vi "Handle WELCOME.vi"(8 "error in (no error)":errorcluster, 9 "WAMP Message":T1 {"Message Codes" items=["HELLO"=1, "WELCOME"=2, "ABORT"=3, "GOODBYE"=6, "ERROR"=8, "PUBLISH"=16, "PUBLISHED"=17, "SUBSCRIBE"=32, "SUBSCRIBED"=33, "UNSUBSCRIBE"=34, "UNSUBSCRIBED"=35, "EVENT"=36, "CALL"=48, "RESULT"=59, "REGISTER"=64, "REGISTERED"=65, "UNREGISTER"=66, "UNREGISTERED"=67, "INVOCATION"=68, "YIELD"=70]}, 11 "WAMP Client in":refnum<class "WAMP Client.lvclass">) -> (0 "error out":errorcluster, 1 "Session ID":u64, 3 "WAMP Client out":refnum<class "WAMP Client.lvclass">)   [LabVIEW 2021, in "wamplv.lvlib" / "WAMP Client.lvclass"]
uses:
  WAMP Client.lvclass
  TypeDef/WAMP Received Message.ctl
  TypeDef/WAMP Message Codes.ctl
  81aa3083-7749-3644-b591-d0aa62dd8321.vi
  <vilib>/JDP Science/JSONtext/JSON text to Variant.vi
  <vilib>/JDP Science/JSONtext/LVClass Serializer/JSONtext LVClass Serializer.lvclass
  WAMP Client.lvclass/WAMP Client.ctl
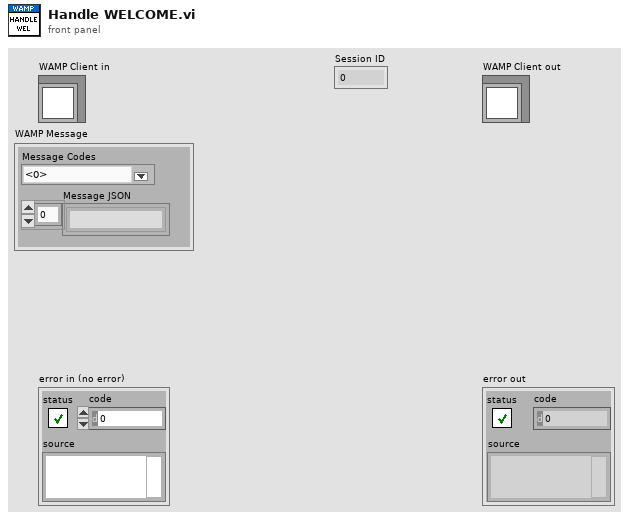
[diagram p1: front panel]
types:
  T1 = typedef "wamplv.lvlib/WAMP Client.lvclass/WAMP Received Message.ctl" = cluster{"Message JSON":string[], "Message Codes":T2}
  T2 = typedef "wamplv.lvlib/WAMP Client.lvclass/WAMP Message Codes.ctl" = u16
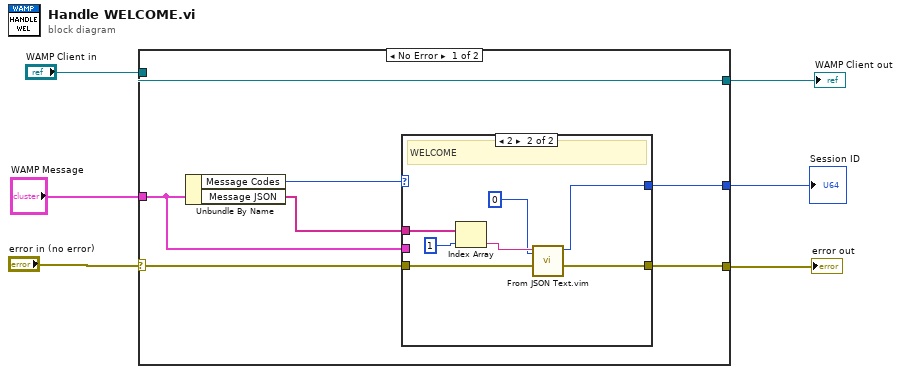
[diagram p0: block diagram]
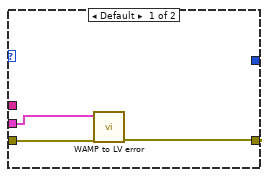
[diagram p2: hidden frame]
diagram:
  n1 = case shown="No Error" "error in (no error)" {
    selector: "error in (no error)" -> [w9 w25]
    tunnel: [w12 w25] -> w5
    tunnel: [w13 w24] -> w3
    tunnel: "WAMP Client in" -> [w13 w24]
    tunnel: [w11 _] -> w2
    tunnel: "WAMP Message" -> [w7 _]
    frame No Error {
      n2 = Unbundle By Name(w7) -> ("Message Codes"=w10:T2, "Message JSON"=w8:string[])
      n3 = case shown="2" w10 {
        tunnel: [w14 w20] -> w12
        tunnel: [_ w19] -> w11
        tunnel: w9 -> [w16 w18]
        tunnel: w8 -> [_ w17]
        tunnel: w7 -> [w15 _]
        frame Default {
          n4 = call "WAMP to LV error.vi"("error in (no error)"=w16, "WAMP Message"=w15) -> ("error out"=w14:errorcluster)  [unwired: 7 in, 2 out]
        }
        frame 2 {
          # "WELCOME"
          n5 = Index Array(array=w17, index=1) -> (element=w22:string)
          n6 = call "From JSON Text.vim"("Data Type and Default Value"=u64 0, "error in (no error)"=w18, "JSON"=w22) -> ("error out"=w20:errorcluster, "Data out"=w19:u64)  [unwired: 7 in]
        }
      }
    }
    frame Error {
    }
  }
  "error out" <- w5
  "WAMP Client out" <- w3
  "Session ID" <- w2
